vi "initSEDSpectrometer.vi"(8 "error in (no error)":errorcluster, 11 "Model in":refnum<class "Model.lvclass">) -> (0 "error out":errorcluster, 1 "Connected":bool, 2 "Device handle":i32, 3 "Model out":refnum<class "Model.lvclass">)   [LabVIEW 2016, in "Model.lvclass"]
uses:
  Model.lvclass
  Model.lvclass/Model.ctl
  ss_sedspectrometer/SEDSpectrometer/SEDSpectrometer.lvclass
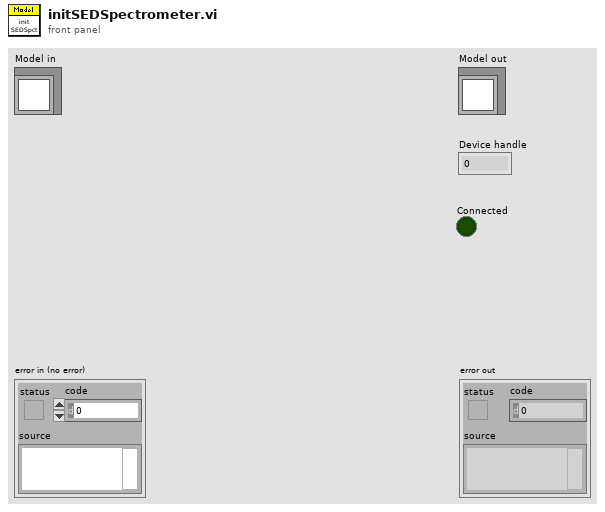
[diagram p1: front panel]
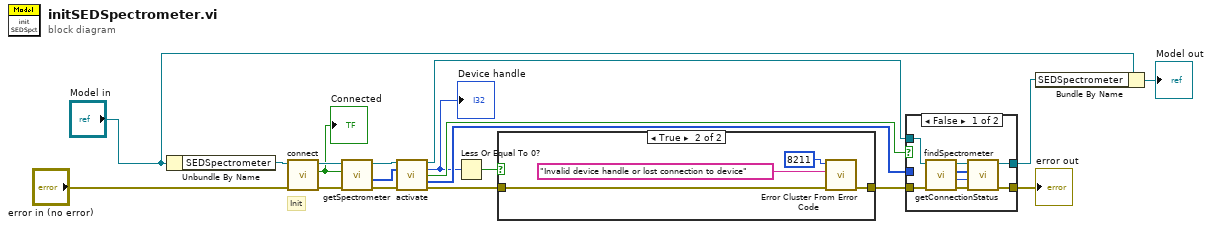
[diagram p0: block diagram]
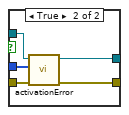
[diagram p3: hidden frame]
diagram:
  # "Init"
  n1 = Unbundle By Name("Model in") -> ("SEDSpectrometer"=w11:refnum<class "SEDSpectrometer.lvclass">)
  n2 = call "connect.vi"("error in (no error)"="error in (no error)", "SEDSpectrometer in"=w11) -> ("error out"=w18:errorcluster, "Connected"=w10:bool, "SEDSpectrometer out"=w19:refnum<class "SEDSpectrometer.lvclass">)  [unwired: 7 in]
  "Connected" <- w10
  n3 = call "getSpectrometer.vi"("error in (no error)"=w18, "Boolean"=w10, "SEDSpectrometer in"=w19) -> ("error out"=w16:errorcluster, "AviableSpec"=w17:u8[], "SEDSpectrometer out"=w15:refnum<class "SEDSpectrometer.lvclass">)  [unwired: 6 in]
  n4 = call "activate.vi"("SEDSpectrometer in"=w15, "DeviceId"=w17, "error in (no error)"=w16) -> ("SEDSpectrometer out"=w14:refnum<class "SEDSpectrometer.lvclass">, "Device handle"=w7:i32, "Activation Error"=w12:bool, "DeviceId"=w13:u8[], "error out"=w5:errorcluster)  [unwired: 8 in]
  "Device handle" <- w7
  n5 = Less Or Equal To 0?(x=w7) -> (x <= 0?=w6:bool)
  n6 = case shown="True" w6 {
    tunnel: w5 -> [w20 w22]
    tunnel: [w20 w21] -> w4
    frame False {
    }
    frame True {
      n7 = call <vilib>:"Error Cluster From Error Code.vi"("error in (no error)"=w22, "error message (\"\")"="Invalid device handle or lost connection to device" ("error message (\"\")"), "error code (0)"=8211) -> ("error out"=w21:errorcluster)  [unwired: 6 in]
    }
  }
  n8 = case shown="False" w12 {
    tunnel: w14 -> [w31 w37]
    tunnel: w4 -> [w30 w36]
    tunnel: [w26 w35] -> w8
    tunnel: w13 -> [_ w34]
    tunnel: [w25 w33] -> w9
    frame False {
      n9 = call "findSpectrometer.vi"("error in (no error)"=w30, "SEDSpectrometer in"=w31) -> ("error out"=w27:errorcluster, "NumOfDevices"=w28:i32, "AviableSpec"=w29:u8[], "SEDSpectrometer out"=w32:refnum<class "SEDSpectrometer.lvclass">)  [unwired: 6 in]
      n10 = call "getConnectionStatus.vi"("SEDSpectrometer in"=w32, "AvailableSpectrometer"=w29, "NumOfDevices"=w28, "error in (no error)"=w27) -> ("SEDSpectrometer out"=w25:refnum<class "SEDSpectrometer.lvclass">, "error out"=w26:errorcluster)  [unwired: 4 in, 1 out]
    }
    frame True {
      n11 = call "activationError.vi"("error in (no error)"=w36, "DeviceId"=w34, "SEDSpectrometer in"=w37) -> ("error out"=w35:errorcluster, "SEDSpectrometer out"=w33:refnum<class "SEDSpectrometer.lvclass">)  [unwired: 6 in, 1 out]
    }
  }
  "error out" <- w8
  n12 = Bundle By Name(cluster="Model in", "SEDSpectrometer"=w9) -> (→"Model out":refnum<class "Model.lvclass">)
